vi "get piece from cube.vi"() -> ()   [LabVIEW 2018]
uses:
  vision/vision info 2.vi
panel:
  out "xx":dbl
  out "_y":dbl
  out "_x":dbl
  in  "move":bool
  in  "speed 1":i32
  in  "step":dbl
  in  "z2":dbl
  in  "z1":dbl
  in  "take":bool
  in  "camera mode":bool
  in  "c2":i8
  in  "c1":i8
  in  "base":i32(slide) scale=-125.0..125.0
  in  "grip":bool
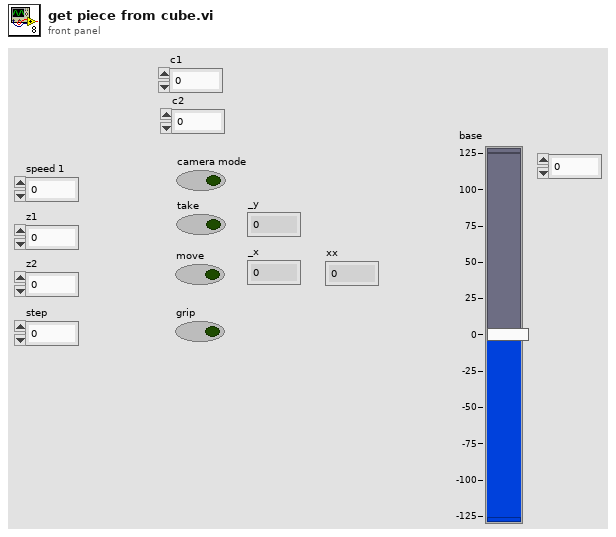
[diagram p1: front panel]
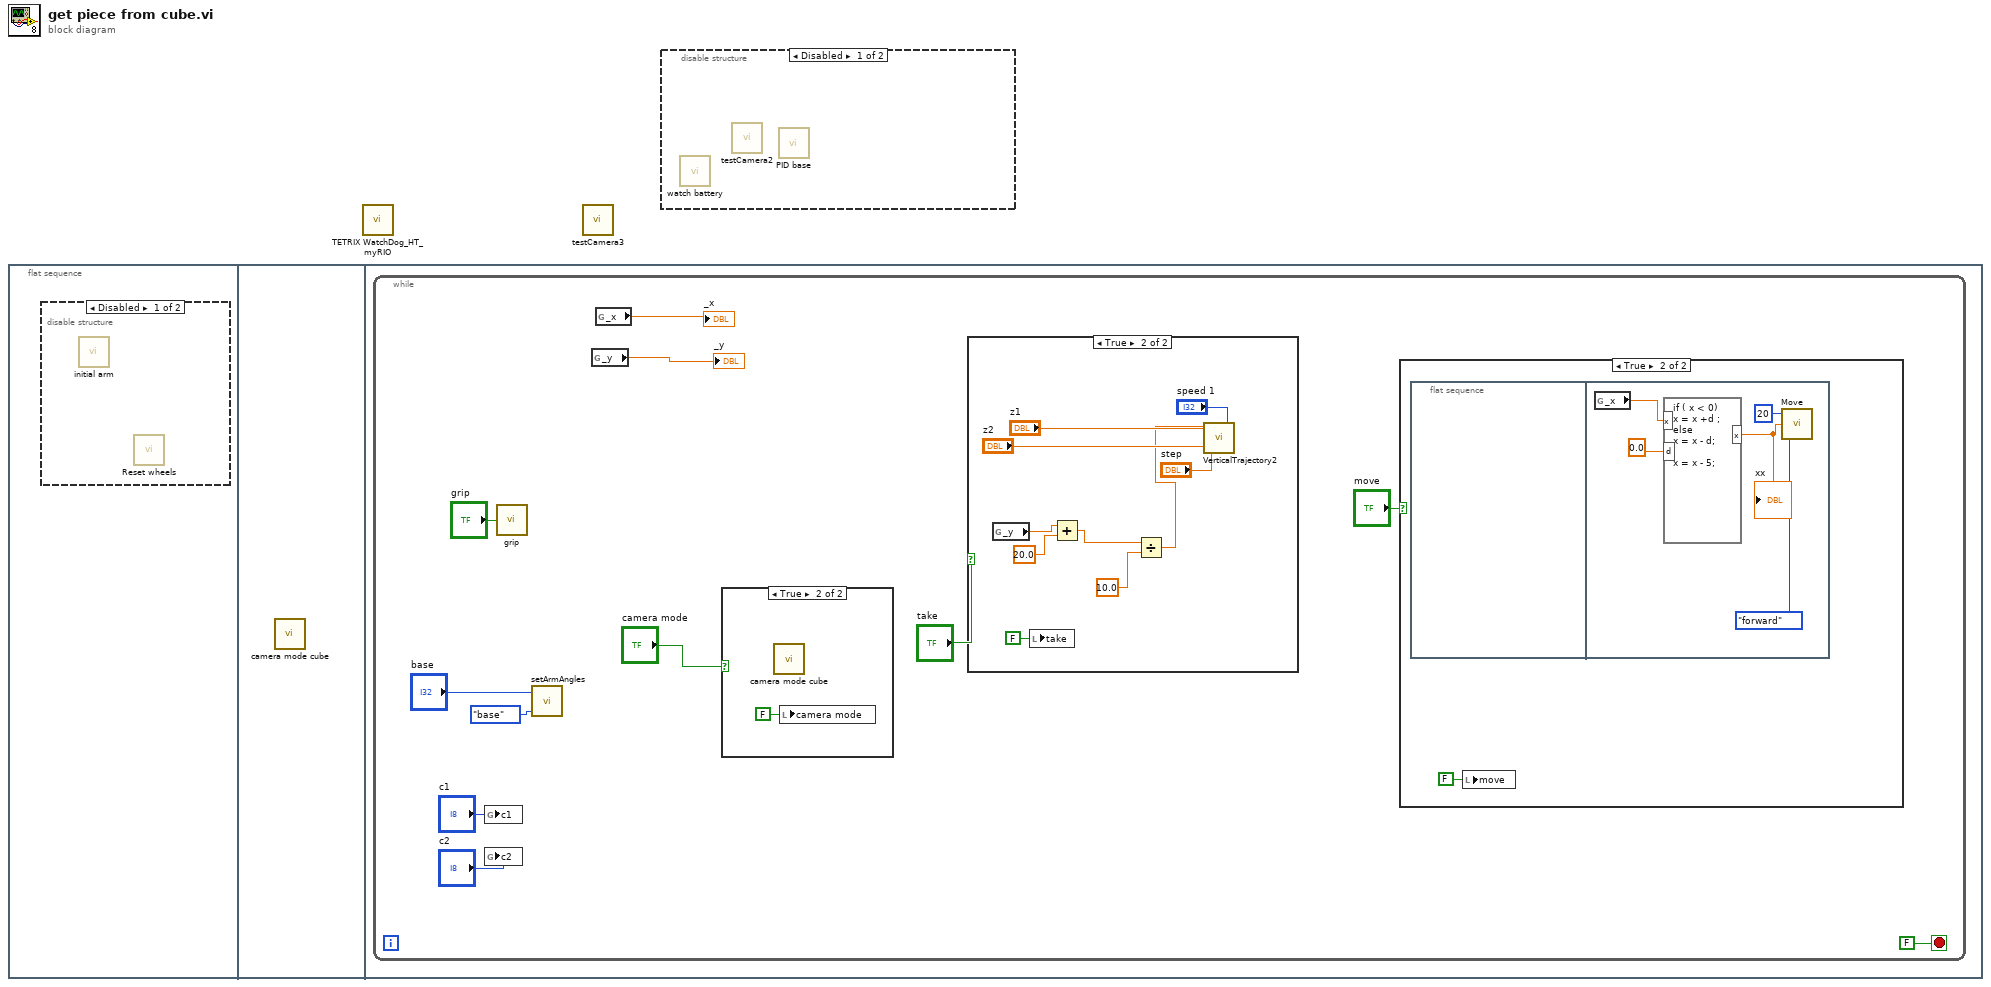
[diagram p0: block diagram]
diagram:
  n1 = flat-sequence {
    frame #0 {
      n2 = disable-structure shown="Disabled" {
        frame Disabled {
          n3 = call "initial arm.vi"() -> ()  [unwired: 12 in]
          n4 = call "Reset wheels.vi"() -> ()  [unwired: 12 in]
        }
        frame Enabled {
        }
      }
    }
    frame #1 {
      n5 = call "camera mode cube.vi"() -> ()  [unwired: 12 in]
    }
    frame #2 {
      n6 = while {
        stop <- FALSE stop-if-true
        n7 = global write "vision info 2.vi" "c1"("c1") -> ()
        n8 = global write "vision info 2.vi" "c2"("c2") -> ()
        n9 = call "grip.vi"("grip"="grip") -> ()
        n10 = call "setArmAngles.vi"("Enum"=enum16{"shoulder", "elbow", "wrist", "base"}."base", "angle"="base") -> ()  [unwired: 2 in]
        n11 = global read "vision info 2.vi" "_y"() -> (→"_y":dbl)
        n12 = global read "vision info 2.vi" "_x"() -> (→"_x":dbl)
        n13 = case shown="True" "camera mode" {
          frame False {
          }
          frame True {
            n14 = call "camera mode cube.vi"() -> ()  [unwired: 12 in]
            n15 = local write "camera mode"(FALSE ("camera mode")) -> ()
          }
        }
        n16 = case shown="True" "take" {
          frame False {
          }
          frame True {
            n17 = global read "vision info 2.vi" "_y"() -> (w20:dbl)
            n18 = local write "take"(FALSE ("take")) -> ()
            n19 = Add(x=w20, y=20.0) -> (x+y=w18:dbl)
            n20 = Divide(x=w18, y=10.0) -> (x/y=w21:dbl)
            n21 = call "VerticalTrajectory2.vi"("speed 1"="speed 1", "step"="step", "z2"="z2", "z1"="z1", "x"=w21) -> ()  [unwired: 3 in]
          }
        }
        n22 = case shown="True" "move" {
          frame False {
          }
          frame True {
            n23 = flat-sequence {
              frame #0 {
              }
              frame #1 {
                n24 = global read "vision info 2.vi" "_x"() -> (w14:dbl)
                n25 = formula code="if ( x < 0)\nx = x +d ;\nelse\nx = x - d;\n\nx = x - 5;"("x"=w14, "d"=0.0 ("dx")) -> ("x"=w13:dbl)
                "xx" <- w13
                n26 = call "Move.vi"("Enum"=enum16{"forward", "backward", "left", "right"}."forward", "distance"=w13, "speed"=20) -> ()  [unwired: 1 in]
              }
            }
            n27 = local write "move"(FALSE ("move")) -> ()
          }
        }
      }
    }
  }
  n28 = call <vilib>:"TETRIX WatchDog_HT_myRIO.vi"() -> ()  [unwired: 3 in, 1 out]
  n29 = call "testCamera3.vi"() -> ()  [unwired: 12 in]
  n30 = disable-structure shown="Disabled" {
    frame Disabled {
      n31 = call "watch battery.vi"() -> ()  [unwired: 12 in]
      n32 = call "testCamera2.vi"() -> ()  [unwired: 12 in]
      n33 = call "PID base.vi"() -> ()  [unwired: 12 in]
    }
    frame Enabled {
    }
  }
